vi "Get Array TD from Element TD.vi"(8 "error in (no error)":errorcluster, 10 "Element Type Descriptor":refnum<class "TypeDescriptor.lvclass">) -> (0 "error out":errorcluster, 2 "Array Type Descriptor":refnum<class "Array.lvclass">)   [LabVIEW 2020, in "lvdata.lvlib" / "type_descriptor.lvlib" / "Array.lvclass"]
uses:
  Type Descriptor Enumeration.ctl
  TypeDescriptor.lvclass/TypeDescriptor.ctl
  Array.lvclass
  Array.lvclass/Array.ctl
  openg_variant.lvlib
  TypeDescriptor.lvclass
  C:/projects/OpenG-Variant-Data-Library/source/library/LVData/Type Descriptor/TypeDescriptor.lvclass
  C:/projects/OpenG-Variant-Data-Library/source/library/Bytes/Bytes.lvclass
  C:/projects/OpenG-Variant-Data-Library/source/library/LVData/Type Descriptor/ArrayTD/Array.lvclass
panel:
  # "Get Array TD from Element TD.vi\n\nReturns the type descriptor of the array element.\n\nPlease visit http://www.OpenG.org to learn about the\nOpen Source LabVIEW software movement.\n\nNOTICE -- YOU MUST LEAVE THIS NOTICE IN PLACE.  PER THE TERMS OF THE LICENSE BELOW, YOU MAY SUBLICENSE THIS SOFTWARE \nIN ANY WAY THAT DOES NOT CONFLICT WITH THIS LICENSE.\n\n### BSD License (http://www.opensource.org/licenses/bsd-license.php) Begin ###\n \nCopyright (c) 2002, Jean-Pierre Drolet <drolet_jp@hotmail.com>\nCopyright (c) 2002-2006, Jim Kring <jim@jimkring.com>\n\nAll rights reserved.\n\nRedistribution and use in source and binary forms, with or without modification, are permitted provided that the following conditions are met:\n\n    * Redistributions of source code must retain the above copyright notice, this list of conditions and the following disclaimer.\n    * Redistributions in binary form must reproduce the above copyright notice, this list of conditions and the following disclaimer in the \n       documentation and/or other materials provided with the distribution.\n    * Neither the name of SciWare, James Kring, Inc., nor the names of its contributors may be used to endorse or promote products derived \n       from this software without specific prior written permission.\n\nTHIS SOFTWARE IS PROVIDED BY THE COPYRIGHT HOLDERS AND CONTRIBUTORS \"AS IS\" AND ANY EXPRESS OR IMPLIED WARRANTIES, \nINCLUDING, BUT NOT LIMITED TO, THE IMPLIED WARRANTIES OF MERCHANTABILITY AND FITNESS FOR A PARTICULAR PURPOSE ARE \nDISCLAIMED. IN NO EVENT SHALL THE COPYRIGHT OWNER OR CONTRIBUTORS BE LIABLE FOR ANY DIRECT, INDIRECT, INCIDENTAL,\n SPECIAL, EXEMPLARY, OR CONSEQUENTIAL DAMAGES (INCLUDING, BUT NOT LIMITED TO, PROCUREMENT OF SUBSTITUTE GOODS OR \nSERVICES; LOSS OF USE, DATA, OR PROFITS; OR BUSINESS INTERRUPTION) HOWEVER CAUSED AND ON ANY THEORY OF LIABILITY, \nWHETHER IN CONTRACT, STRICT LIABILITY, OR TORT (INCLUDING NEGLIGENCE OR OTHERWISE) ARISING IN ANY WAY OUT OF THE USE \nOF THIS SOFTWARE, EVEN IF ADVISED OF THE POSSIBILITY OF SUCH DAMAGE.\n\n### BSD License End ###"
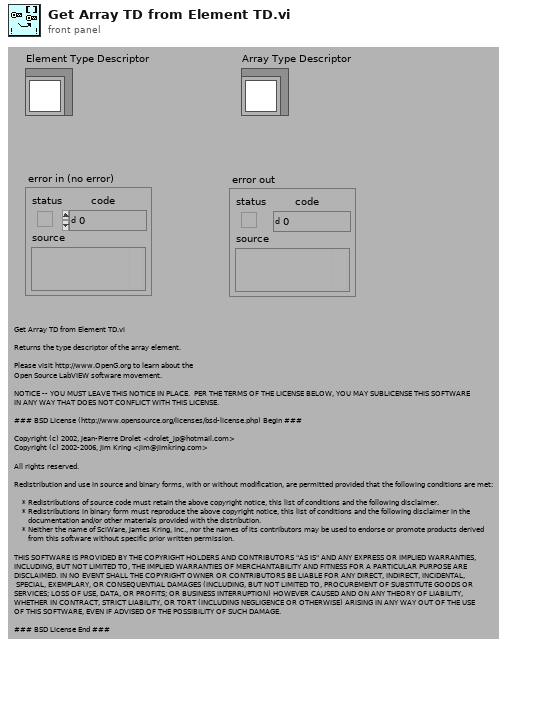
[diagram p1: front panel]
types:
  T1 = typedef "openg_variant.lvlib/Type Descriptor Enumeration.ctl" = enum8{"<Null>", "I8", "I16", "I32", "I64", "U8", "U16", "U32", "U64", "SGL", "DBL", "EXT", "CSG", "CDB", "CXT", "0x0F", "0x10", "0x11", "0x12", "0x13", "0x14", "Enum U8", "Enum U16", "Enum U32", "Enum U64", "SGL PQ", "DBL PQ", "EXT PQ", "CSG PQ", "CDB PQ", "CXT PQ", "0x1F", "0x20", "Boolean", "0x22", "0x23", "0x24", "0x25", "0x26", "0x27", "0x28", "0x29", "0x2A", "0x2B", "0x2C", "0x2D", "0x2E", "0x2F", "String", "0x31", "Path", "Pict", "0x34", "0x35", "0x36", "DAQ", "0x38", "0x39", "0x3A", "0x3B", "0x3C", "0x3D", "0x3E", "0x3F", "Array", "0x41", "0x42", "0x43", "0x44", "0x45", "0x46", "0x47", "0x48", "0x49", "0x4A", "0x4B", "0x4C", "0x4D", "0x4E", "0x4F", "Cluster", "0x51", "0x52", "Variant", "Waveform", "0x55", "0x56", "0x57", "0x58", "0x59", "0x5A", "0x5B", "0x5C", "0x5D", "0x5E", "Fixed Point", "0x60", "0x61", "0x62", "0x63", "0x64", "0x65", "0x66", "0x67", "0x68", "0x69", "0x6A", "0x6B", "0x6C", "0x6D", "0x6E", "0x6F", "Refnum", "0x71", "0x72", "Set Collection", "Map Collection"}
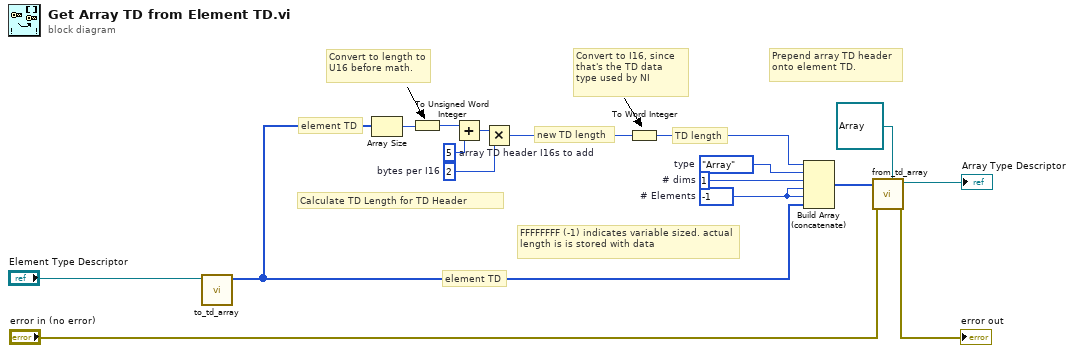
[diagram p0: block diagram]
diagram:
  w16 = u16 2  # bytes per I16
  w14 = u16 5  # array TD header I16s to add
  w10 = i16 1  # # dims
  w9 = i16 -1  # # Elements
  w8 = Type_Descriptor_Enumeration."Array"  # type
  # "FFFFFFFF (-1) indicates variable sized. actual length is is stored with data"
  # "TD length"
  # "Calculate TD Length for TD Header"
  # "element TD"
  # "Prepend array TD header onto element TD."
  # "element TD"
  # "new TD length"
  # "Convert to I16, since that's the TD data type used by NI"
  # "Convert to length to U16 before math."
  n1 = call "to_td_array.vi"("TypeDescriptor in"="Element Type Descriptor") -> ("type string"=w6:i16[])  [unwired: 10 in]
  n2 = Array Size(array=w6) -> (size(s)=w11:i32)
  n3 = To Unsigned Word Integer(number=w11) -> (unsigned 16bit integer=w13:u16)
  n4 = Add(x=w13, y=w14) -> (x+y=w15:u16)
  n5 = Multiply(x=w15, y=w16) -> (x*y=w17:u16)
  n6 = To Word Integer(number=w17) -> (16bit integer=w12:i16)
  n7 = Build Array (concatenate)(w12, w8, w10, w9, w9, w6) -> (w5:i16[])
  n8 = call "from_td_array.vi"("type"=refnum<class "Array.lvclass"> refnum ("Array Type Descriptor"), "error in"="error in (no error)", "type descriptor array"=w5) -> ("error out"=→"error out":errorcluster, "TypeDescriptor out"=→"Array Type Descriptor":refnum<class "Array.lvclass">)  [unwired: 7 in]
